vi "camera-write_exposure-auto.vi"(6 "error in (no error)":errorcluster, 8 "Option":enum16{"Off", "Once", "Continuous", "Stop"}(ring), 9 "IMAQ Session In":refnum<k11>) -> (0 "error out":errorcluster, 1 "Data":string, 2 "Address":string, 3 "IMAQ Session Out":refnum<k11>)   [LabVIEW 2012]
panel:
  out "Loop Iteration":i32
  out "ACK/NAK":string
  out "String to Write":string
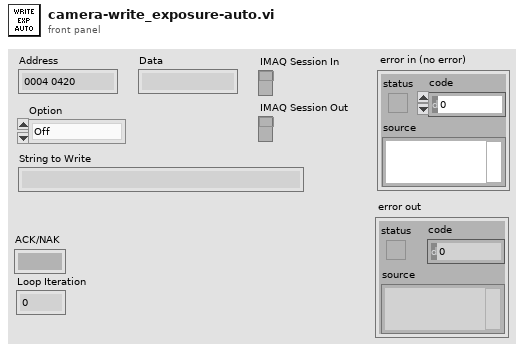
[diagram p1: front panel]
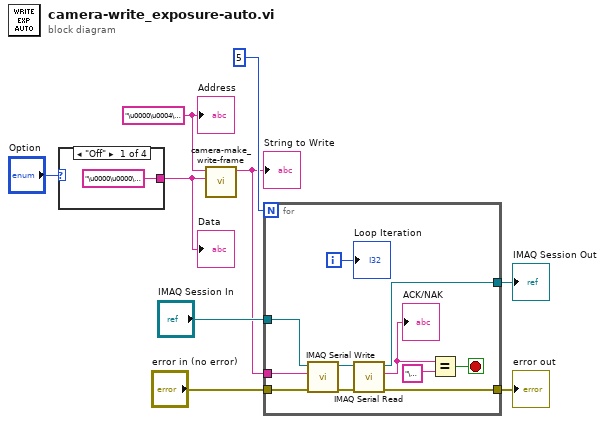
[diagram p0: block diagram]
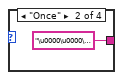
[diagram p2: hidden frame]
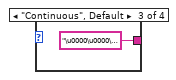
[diagram p3: hidden frame]
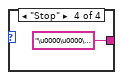
[diagram p4: hidden frame]
diagram:
  w9 = "\u0000\u0004\u0004 " ("Address")
  n1 = case shown="\"Off\"" "Option" {
    tunnel: ["\u0000\u0000\u0000\u0000" ("Address") "\u0000\u0000\u0000\u0001" ("Address") "\u0000\u0000\u0000\u0002" ("Address") "\u0000\u0000\u0000\u0003" ("Address")] -> w7
    frame "Off" {
    }
    frame "Once" {
    }
    frame "Continuous", Default {
    }
    frame "Stop" {
    }
  }
  "Data" <- w7
  n2 = call "camera-make_write-frame.vi"("Data"=w7, "Address"=w9) -> ("Serial String"=w4:string)  [unwired: 9 in]
  "String to Write" <- w4
  n3 = for {
    N: 5 -> [_]
    tunnel: "IMAQ Session In" -> [w24]
    tunnel: w4 -> [w23]
    tunnel: [w22] -> w3
    tunnel: "error in (no error)" -> [w21]
    tunnel: [w19] -> w1
    i -> [w15]
    stop <- w18 stop-if-true
    n4 = call <vilib>:"IMAQ Serial Write.vi"("error in (no error)"=w21, "String to write"=w23, "IMAQ Session In"=w24) -> ("error out"=w20:errorcluster, "IMAQ Session Out"=w14:refnum<k11>)  [unwired: 5 in]
    n5 = call <vilib>:"IMAQ Serial Read.vi"("error in (no error)"=w20, "IMAQ Session In"=w14) -> ("error out"=w19:errorcluster, "String Read"=w17:string, "IMAQ Session Out"=w22:refnum<k11>)  [unwired: 4 in, 1 out]
    "ACK/NAK" <- w17
    n6 = Equal?(x=w17, y="\u0006") -> (x = y?=w18:bool)
    "Loop Iteration" <- w15
  }
  "IMAQ Session Out" <- w3
  "error out" <- w1
  "Address" <- w9
